vi "PantherLAB_log - Add Helper Loop to DQMH Module.vi"(10 "Helper Loop Name":string, 11 "Module Info":T1) -> (0 "error out":errorcluster)   [LabVIEW 2016]
doc: "_____\nCreated using DQMH Framework: Event Scripter 7.1.0.1450."
uses:
  <vilib>/Delacor/Delacor QMH/Libraries/_Scripting Support/Module Info--cluster.ctl
  <vilib>/Delacor/Delacor QMH/Libraries/_Scripting Support/Module Type--enum.ctl
  PantherLAB Scripting Hooks/PantherLAB_Scripting.lvlib
  <vilib>/Delacor/Delacor QMH/Libraries/_Scripting Support/dqmh_lib_DQMH Scripting Support.lvlib
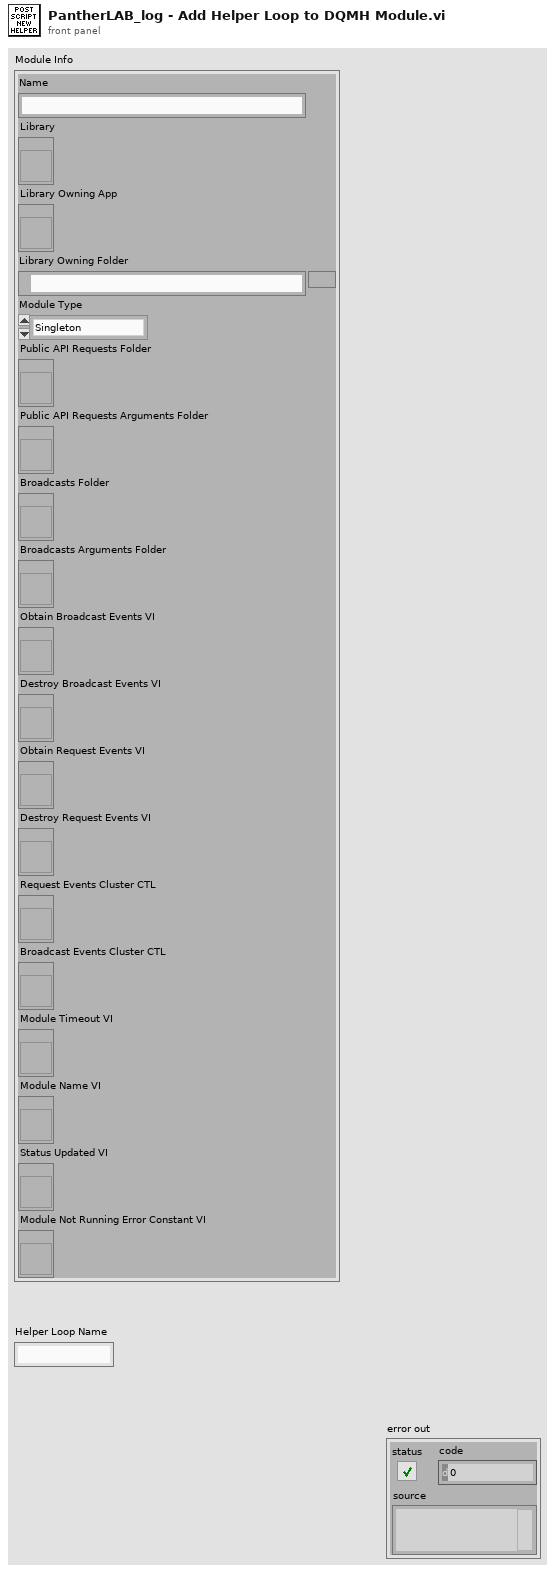
[diagram p1: front panel]
types:
  T1 = typedef "dqmh_lib_DQMH Scripting Support.lvlib/Module Info--cluster.ctl" = cluster{"Name":string, "Library":refnum<vi>, "Library Owning App":refnum<vi>, "Library Owning Folder":path, "Module Type":T2, "Public API Requests Folder":refnum<vi>, "Public API Requests Arguments Folder":refnum<vi>, "Broadcasts Folder":refnum<vi>, "Broadcasts Arguments Folder":refnum<vi>, "Obtain Broadcast Events VI":refnum<vi>, "Destroy Broadcast Events VI":refnum<vi>, "Obtain Request Events VI":refnum<vi>, "Destroy Request Events VI":refnum<vi>, "Request Events Cluster CTL":refnum<vi>, "Broadcast Events Cluster CTL":refnum<vi>, "Module Timeout VI":refnum<vi>, "Module Name VI":refnum<vi>, "Status Updated VI":refnum<vi>, "Module Not Running Error Constant VI":refnum<vi>}
  T2 = typedef "dqmh_lib_DQMH Scripting Support.lvlib/Module Type--enum.ctl" = enum16{"Singleton", "Cloneable"}
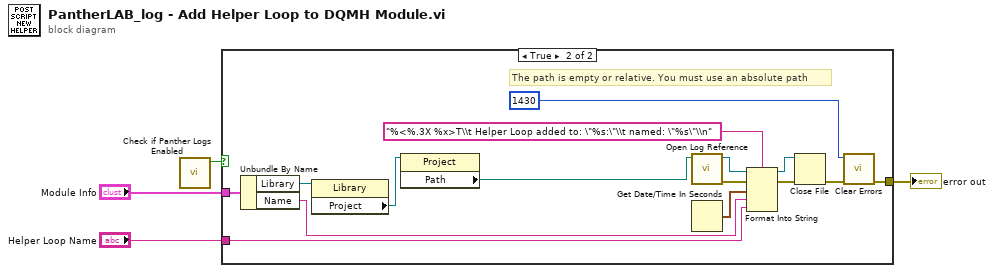
[diagram p0: block diagram]
diagram:
  n1 = call "Check if Panther Logs Enabled.vi"() -> ("PantherLogs Enabled?"=w3:bool)  [unwired: 11 in]
  n2 = case shown="True" w3 {
    tunnel: [_ w16] -> w4
    tunnel: "Module Info" -> [_ w15]
    tunnel: "Helper Loop Name" -> [_ w7]
    frame False {
    }
    frame True {
      # "The path is empty or relative. You must use an absolute path"
      n3 = Unbundle By Name(w15) -> ("Library"=w14:refnum<vi>, "Name"=w8:string)
      n4 = property class="Library"(reference=w14) -> ("Project"=w13:refnum<vi>)  [unwired: 1 in, 2 out]
      n5 = property class="Project"(reference=w13) -> ("Path"=w9:path)  [unwired: 1 in, 2 out]
      n6 = call "Open Log Reference.vi"("Project Path"=w9) -> ("error out"=w19:errorcluster, "File Reference"=w12:refnum<file>)  [unwired: 9 in]
      n7 = Get Date/Time In Seconds() -> (seconds since 1Jan1904=w10:timestamp)
      n8 = Format Into String(format string="%<%.3X %x>T\\t Helper Loop added to: \"%s:\"\\t named: \"%s\"\\n", initial string=w12, error in=w19, w10, w8, w7) -> (resulting string=w11:refnum<file>, error out=w18:errorcluster)
      n9 = Close File(refnum=w11, error in=w18) -> (error out=w17:errorcluster)  [unwired: 1 out]
      n10 = call <vilib>:"Clear Errors.vi"("error in (no error)"=w17, "specific error code to clear (0: all)"=1430) -> ("error out"=w16:errorcluster)  [unwired: 4 in, 1 out]
    }
  }
  "error out" <- w4
